vi "Read #cars owned.vi"(8 "error in (no error)":errorcluster, 11 "Michael Jordan in":refnum<class "Michael Jordan.lvclass">) -> (0 "error out":errorcluster, 2 "#cars owned":i16, 3 "Michael Jordan out":refnum<class "Michael Jordan.lvclass">)   [LabVIEW 2019, in "Michael Jordan.lvclass"]
uses:
  Michael Jordan.lvclass
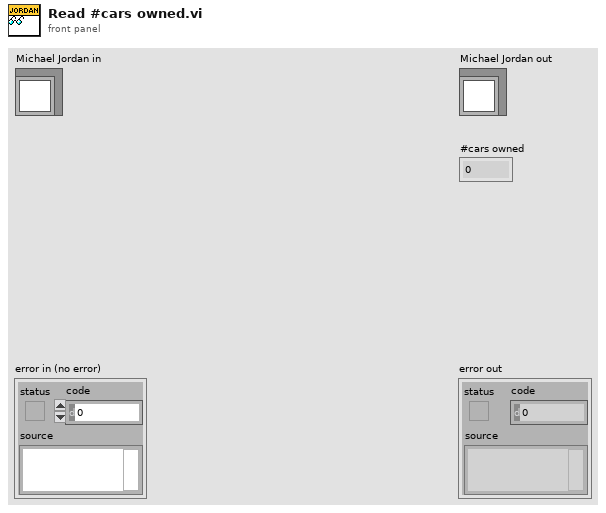
[diagram p1: front panel]
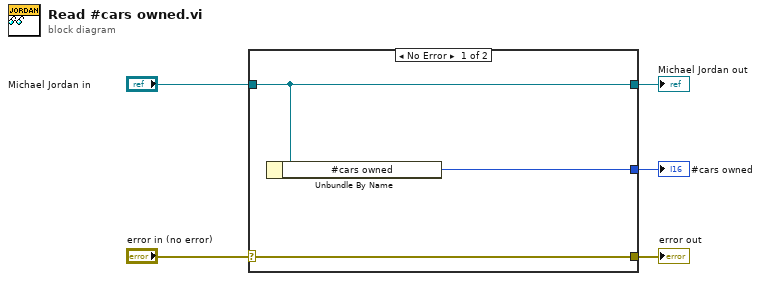
[diagram p0: block diagram]
diagram:
  n1 = case shown="No Error" "error in (no error)" {
    selector: "error in (no error)" -> [w8 w9]
    tunnel: [w8 w9] -> w4
    tunnel: [w7 w10] -> w2
    tunnel: "Michael Jordan in" -> [w7 w10]
    tunnel: [w6 _] -> w1
    frame No Error {
      n2 = Unbundle By Name(w7) -> ("#cars owned"=w6:i16)
    }
    frame Error {
    }
  }
  "error out" <- w4
  "Michael Jordan out" <- w2
  "#cars owned" <- w1
